vi "Recieve.vi"(8 "error in (no error)":errorcluster, 10 "Dropped?":bool, 11 "Response Core in":refnum<class "Interruptible Reply Core.lvclass">) -> (0 "error out":errorcluster, 1 "Success?":bool, 3 "Data":refnum<class "Data.lvclass">)   [LabVIEW 2020, in "Publisher.lvlib" / "Interruptible Reply Core.lvclass"]
doc: "Await the response from the sent message. Also terminates the Listen for Interrupt method when the sent message responds.\n\nThis implementation dequeues a Data element and then drops the core returning the Data."
uses:
  Interruptible Reply Core.lvclass
  PPL/HDH.Data.Generic.lvlibp/Data.lvclass
  Interruptible Reply Core.lvclass/Interruptible Reply Core.ctl
  PPL/HDH.Data.Generic.lvlibp/Synchronization/Queue/Queue.lvclass
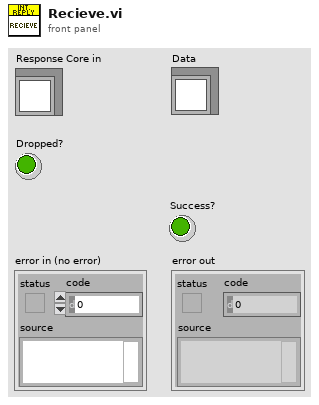
[diagram p1: front panel]
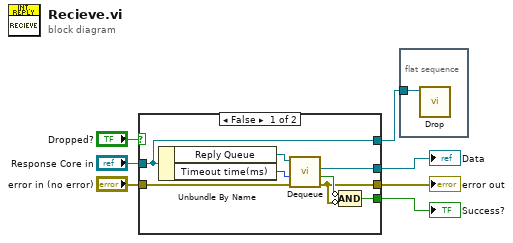
[diagram p0: block diagram]
diagram:
  n1 = case shown="False" "Dropped?" {
    tunnel: "Response Core in" -> [w8 w16]
    tunnel: [w10 w17] -> w1
    tunnel: "error in (no error)" -> [w13 w17]
    tunnel: [w12 _] -> w5
    tunnel: [w9 _] -> w4
    tunnel: [w8 w16] -> w2
    frame False {
      n2 = Unbundle By Name(w8) -> ("Reply Queue"=w15:refnum<class "Queue.lvclass">, "Timeout time(ms)"=w14:i32)
      n3 = call "Dequeue.vi"("error in (no error)"=w13, "timeout in ms (-1)"=w14, "Queue in"=w15) -> ("error out"=w10:errorcluster, "timed out?"=w11:bool, "Data"=w12:refnum<class "Data.lvclass">)  [unwired: 5 in, 1 out]
      n4 = Compound Arithmetic op=AND(invert w11, invert w10) -> (w9:bool)
    }
    frame True {
    }
  }
  "error out" <- w1
  "Data" <- w5
  "Success?" <- w4
  n5 = flat-sequence {
    tunnel: w2 -> [w18]
    frame #0 {
      n6 = call-dynamic "Drop.vi"("Response Core in"=w18) -> ()  [unwired: 11 in]
    }
  }
